vi "SUB_COM1_ESC3_ChkDbgMask_new.vi"(3 "VISA resource name":refnum<visa-resource-name>) -> (0 "MSG OUT":string, 1 "duplicate VISA OUT":refnum<visa-resource-name>)   [LabVIEW 2011]
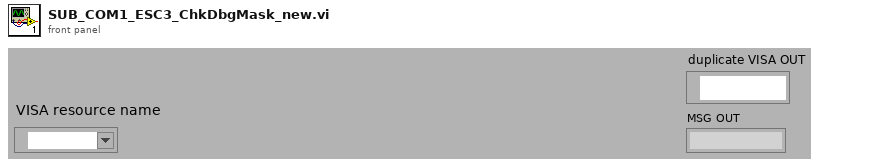
[diagram p1: front panel]
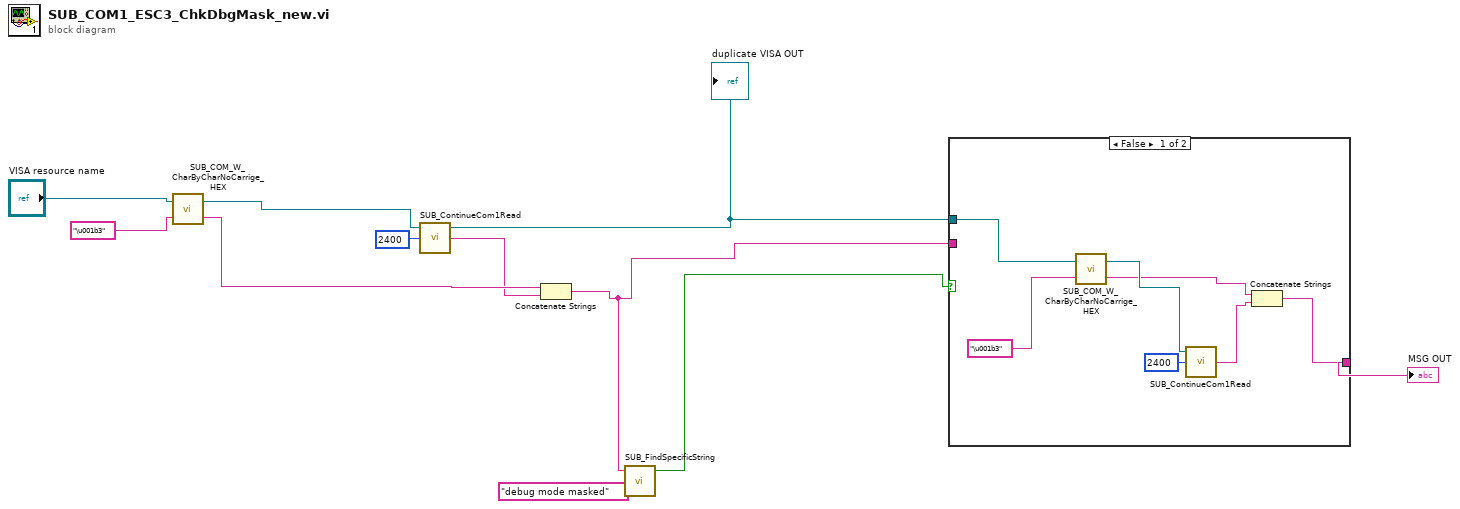
[diagram p0: block diagram]
diagram:
  n1 = call "SUB_COM_W_CharByCharNoCarrige_HEX.vi"("cmd string"="\u001b3" ("write buffer"), "duplicate VISA resource name"="VISA resource name") -> ("OUT string"=w3:string, "VISA resource OUT"=w4:refnum<visa-resource-name>)
  n2 = call "SUB_ContinueCom1Read.vi"("Numeric"=2400, "duplicate VISA resource name 2"=w4) -> ("String"=w2:string, "duplicate VISA resource name"=w8:refnum<visa-resource-name>)  [unwired: 1 in, 1 out]
  "duplicate VISA OUT" <- w8
  n3 = Concatenate Strings(w3, w2) -> (w1:string)
  n4 = call "SUB_FindSpecificString.vi"("Find this String"="debug mode masked", "String data"=w1) -> ("Found"=w9:bool)  [unwired: 2 in, 1 out]
  n5 = case shown="False" w9 {
    tunnel: w8 -> [w17 _]
    tunnel: [w12 w19] -> w7
    tunnel: w1 -> [_ w19]
    frame False {
      n6 = call "SUB_COM_W_CharByCharNoCarrige_HEX.vi"("cmd string"="\u001b3" ("write buffer"), "duplicate VISA resource name"=w17) -> ("OUT string"=w14:string, "VISA resource OUT"=w15:refnum<visa-resource-name>)
      n7 = call "SUB_ContinueCom1Read.vi"("Numeric"=2400, "duplicate VISA resource name 2"=w15) -> ("String"=w13:string)  [unwired: 1 in, 2 out]
      n8 = Concatenate Strings(w14, w13) -> (w12:string)
    }
    frame True {
    }
  }
  "MSG OUT" <- w7
